vi "Target-Scoped FIFO (1xI16) - Write.vi"(0 "data in":T1, 2 "reset":bool, 5 "input valid":bool, 9 "write enable (T)":bool=TRUE, 11 "Target-Scoped FIFO (1xI16)":T2) -> (14 "ready for input":bool, 15 "fifo full":bool)   [LabVIEW 2018, in "Streaming FPGA.lvlib"]
doc: "Writes a Target-scoped FIFO using the data type provided by the <B>Data Type (1xI16).ctl</B>.\n\nUse the <B>write enable</B> input to enable or disable the FIFO writing. <B>fifo full</B> is true if the FIFO was full in the previous clock cycle."
uses:
  Streaming FPGA.lvlib
  Data Type (1xI16).ctl
  Target-Scoped FIFO (1xI16) Resource.ctl
  <vilib>/rvi/DataTransferAndStorage/Container/Common/niFpgaContainerExecOnDevCompGetState.vi
  <vilib>/rvi/Emulation/niFpgaEmulationIsFPGAContextNoSignature.vi
  <vilib>/rvi/Emulation/niFpgaSctlEmulationGetInTimedLoop.vi
  <vilib>/rvi/errors/niFpgaSetErrorForExecOnDevCompSimple.vi
  <vilib>/rvi/eio/common/nirviEmuReportErrorAndStop.vi
  <vilib>/rvi/DataTransferAndStorage/Container/Common/niFpgaContainerGetUniqueNameForEmu.vi
  <vilib>/rvi/FIFO/Fifo_Resource/nirvififoEmulationSetSize.vi
  <vilib>/rvi/FIFO/Fifo_Resource/nirviFifoEmulationQueueMgr.vi
  <instcachedir>/0/nirviFifoEmulationQueueMgr_E5CAEC123FF24DC58D834DCA3CDAA9B5.lvgen/nirviFifoEmulationQueueMgr_E5CAEC123FF24DC58D834DCA3CDAA9B5_043.vi
  <vilib>/rvi/FIFO/Fifo_Resource/nirvififoEmulationDetermineInputValidOut.vi
  <vilib>/rvi/FIFO/Fifo_Resource/nirvififoEmulationCreateLock.vi
  <vilib>/rvi/Emulation/niFpgaProcessEmulError.vi
  <vilib>/rvi/FIFO/Fifo_Resource/nirvififoEmulationObtainLock.vi
  <vilib>/rvi/FIFO/Fifo_Resource/nirvififoEmulationReleaseLock.vi
  <vilib>/rvi/occurrence/nirviWaitOnOccurrenceBase.vi
  <vilib>/rvi/errors/nirviReportUnexpectedCaseInternalError.vi
  <vilib>/rvi/errors/nirviReportUnexpectedCaseInternalError (U32).vi
  <vilib>/Utility/error.llb/Clear Errors.vi
  <vilib>/rvi/interface/RandomDataEmulation/niFpgaRandomDataHandleErrors.vi
  <vilib>/rvi/DataTransferAndStorage/Container/XNode/niFpgaContainer.xnode
  <vilib>/rvi/FIFO/Fifo_Resource/niFpgaFifoEmulationRefIn.vi
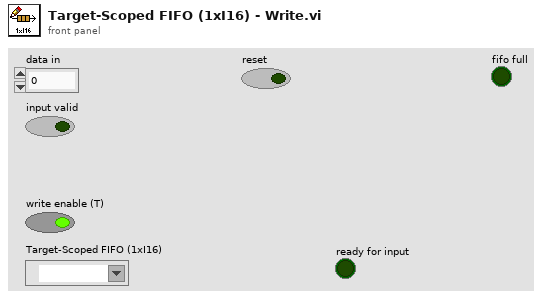
[diagram p1: front panel]
types:
  T1 = typedef "Streaming FPGA.lvlib/Data Type (1xI16).ctl" = i16
  T2 = typedef "Streaming FPGA.lvlib/Target-Scoped FIFO (1xI16) Resource.ctl" = refnum<k21>
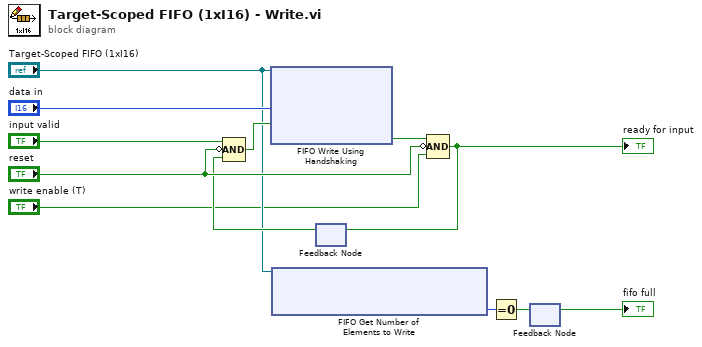
[diagram p0: block diagram]
diagram:
  n1 = xnode "FIFO Get Number of Elements to Write"("FIFO In"="Target-Scoped FIFO (1xI16)") -> ("Number of Elements to Write"=w5:u32)  [unwired: 1 out]
  n2 = feedback #1() -> (w7:bool)  [unwired: 1 in]
  n3 = Compound Arithmetic op=AND("input valid", invert "reset", w7) -> (w10:bool)
  n4 = xnode "FIFO Write Using Handshaking"("Element"="data in", "Input Valid"=w10, "FIFO In"="Target-Scoped FIFO (1xI16)") -> ("Ready for Input"=w12:bool)  [unwired: 1 out]
  n5 = Compound Arithmetic op=AND(w12, invert "reset", "write enable (T)") -> (w8:bool)
  "ready for input" <- w8
  n6 = feedback-in #1(w8) -> ()
  n7 = Equal To 0?(x=w5) -> (x = 0?=w4:bool)
  n8 = feedback-in #2(w4) -> ()
  n9 = feedback #2() -> (→"fifo full":bool)  [unwired: 1 in]
